vi "PicoScope2000aGetValuesOverlappedBulk.vi"(5 "Segment Range":T1 {"toSegmentIndex" format="%.4p"; "fromSegmentIndex" format="%.4p"}, 7 "Buffer and Transfer Settings":T2={"startIndex"=0, "Samples"=1000, "Down Sample Ratio"=1, "Down-Sample Mode"=1} {"Down-Sample Mode" items=["None"=2147483648, "Aggregate"=1, "Decimate"=2, "Average"=4]; "Down Sample Ratio" step=1; "Samples" format="%_6p"}, 8 "error in (no error)":errorcluster, 11 "handle in":i16) -> (0 "error out":errorcluster, 3 "handle out":i16, 4 "Pointer to Overflow":u64[](array[numeric]), 6 "noOfSamples":u64)   [LabVIEW 2010]
doc: "Calls GetValuesOverlappedBulk"
uses:
  ps2000a.dll
  shared/Buffer and Transfer Settings.ctl
  shared/Segment Range.ctl
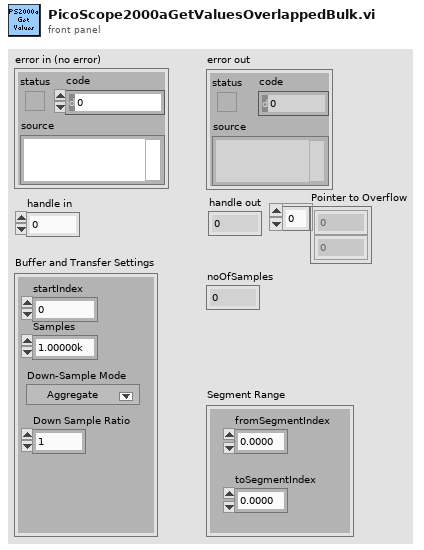
[diagram p1: front panel]
types:
  T1 = typedef "Segment Range.ctl" = cluster{"fromSegmentIndex":u64, "toSegmentIndex":u64}
  T2 = typedef "Buffer and Transfer Settings.ctl" = cluster{"startIndex":u64, "Samples":u64, "Down Sample Ratio":u64, "Down-Sample Mode":u32}
  T3 = cluster{"status":bool, "code":u32, "source":string}
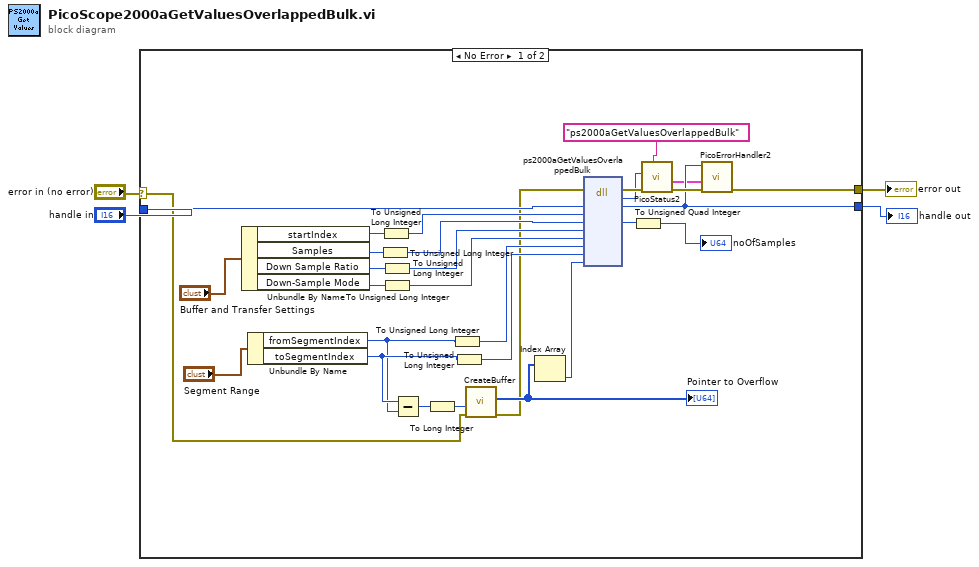
[diagram p0: block diagram]
diagram:
  n1 = case shown="No Error" "error in (no error)" {
    selector: "error in (no error)" -> [w7 w35]
    tunnel: "handle in" -> [w25 w36]
    tunnel: [w28 w36] -> w4
    tunnel: [w31 w35] -> w3
    frame No Error {
      n2 = Unbundle By Name("Buffer and Transfer Settings") -> ("startIndex"=w20:u64, "Samples"=w18:u64, "Down Sample Ratio"=w17:u64, "Down-Sample Mode"=w16:u32)
      n3 = Unbundle By Name("Segment Range") -> ("fromSegmentIndex"=w23:u64, "toSegmentIndex"=w24:u64)
      n4 = To Unsigned Long Integer(number=w18) -> (unsigned 32bit integer=w15:u32)
      n5 = To Unsigned Long Integer(number=w20) -> (unsigned 32bit integer=w19:u32)
      n6 = To Unsigned Long Integer(number=w17) -> (unsigned 32bit integer=w14:u32)
      n7 = To Unsigned Long Integer(number=w16) -> (unsigned 32bit integer=w13:u32)
      n8 = Subtract(x=w24, y=w23) -> (x-y=w26:u64)
      n9 = To Long Integer(number=w26) -> (32bit integer=w9:i32)
      n10 = To Unsigned Long Integer(number=w23) -> (unsigned 32bit integer=w22:u32)
      n11 = To Unsigned Long Integer(number=w24) -> (unsigned 32bit integer=w21:u32)
      n12 = call "CreateBuffer.vi"("error in (no error)"=w7, "Buffer size"=w9) -> ("error out"=w8:errorcluster, "Pointer and BufferSize"=w10:u64[])  [unwired: 8 in]
      "Pointer to Overflow" <- w10
      n13 = Index Array(array=w10) -> (element=w6:u64)  [unwired: 1 in]
      n14 = dll-call lib="ps2000a.dll" fn="ps2000aGetValuesOverlappedBulk" ("ps3000.dll:_ps3000_open_unit@0")(error in=w8, "handle"=w25, "startIndex"=w19, "noOfSamples"=w15, "downSampleRatio"=w14, "downSampleRatioMode"=w13, "fromSegmentIndex"=w22, "toSegmentIndex"=w21, "overflow"=w6) -> (error out=w29:errorcluster, "PICO_STATUS"=w27:u32, "handle"=w28:i16, "noOfSamples"=w11:u32)  [unwired: 8 in, 1 out]
      n15 = To Unsigned Quad Integer(1:w11) -> (0:→"noOfSamples":u64)
      n16 = call "PicoStatus2.vi"("PICO source"="ps2000aGetValuesOverlappedBulk" ("source"), "Error in"=w29, "PICO STATUS"=w27) -> ("error out"=w34:errorcluster, "PICO_STATUS out"=w5:T3)  [unwired: 5 in]
      n17 = call "PicoErrorHandler2.vi"("error in (no error)"=w34, "PICO_STATUS in"=w5, "handle In"=w28) -> ("error out"=w31:errorcluster)  [unwired: 8 in]
    }
    frame Error {
    }
  }
  "error out" <- w3
  "handle out" <- w4
